vi "Write Image Type.vi"(11 "Output Image Type":T1) -> ()   [LabVIEW 2020, in "SimpleDependencyInspector.lvlib"]
uses:
  Image Type--enum.ctl
  <resource>/dialog/lvconfig.llb/LV Config Write Numeric (I32).vi
  SimpleDependencyInspector.lvlib
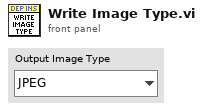
[diagram p1: front panel]
types:
  T1 = typedef "SimpleDependencyInspector.lvlib/Image Type--enum.ctl" = enum16{"JPEG", "PNG", "BMP", "SVG"}
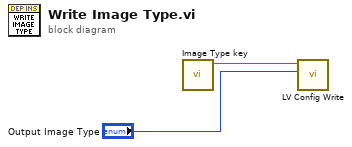
[diagram p0: block diagram]
diagram:
  n1 = call "Image Type key.vi"() -> ("String"=w2:string)  [unwired: 11 in]
  n2 = call-poly <resource>:"LV Config Write.vi"("value"="Output Image Type", "key"=w2) -> ()  [unwired: 5 in, 1 out]
